vi "_Simple_Demo.vi"() -> ()   [LabVIEW 2017]
panel:
  out "Data":dbl(graph)
  out "Image":picture
  in  "stop":bool
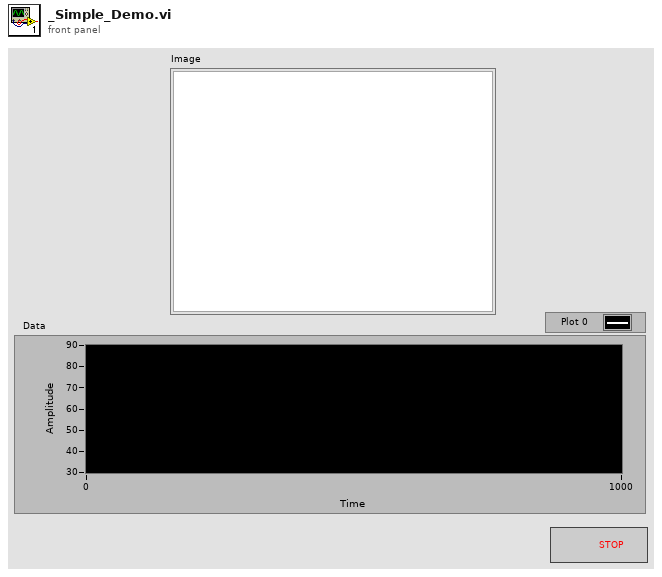
[diagram p1: front panel]
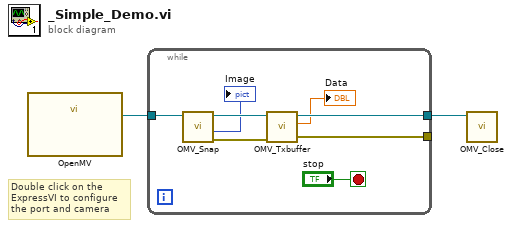
[diagram p0: block diagram]
diagram:
  # "Double click on the \nExpressVI to configure\nthe port and camera"
  n1 = call "OpenMV"() -> ("USB Connection out"=w1:refnum<visa-resource-name>)
  n2 = while {
    tunnel: w1 -> [w10]
    tunnel: [w8] -> w2
    tunnel: [w4] -> _
    stop <- "stop" stop-if-true
    n3 = call <userlib>:"OMV_Snap.vi"("VISA Refnum in"=w10) -> ("error out"=w5:errorcluster, "picture"=→"Image":picture, "VISA Refnum out"=w9:refnum<visa-resource-name>)  [unwired: 7 in, 1 out]
    n4 = call <userlib>:"OMV_Txbuffer.vi"("error in (no error)"=w5, "VISA Refnum in"=w9) -> ("error out"=w4:errorcluster, "Data"=→"Data":dbl, "VISA Refnum out"=w8:refnum<visa-resource-name>)  [unwired: 7 in]
  }
  n5 = call <userlib>:"OMV_Close.vi"("VISA Refnum in"=w2) -> ()  [unwired: 11 in]
